vi "CRYGet Max Size.vi"(10 "Value Rows":i32[](array[numeric]), 11 "Curve Rows":i32[](array[numeric])) -> (3 "Max Size":i32)   [LabVIEW 2013]
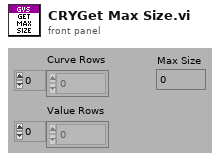
[diagram p1: front panel]
types:
  T1 = typedef "CRYData Cluster.ctl" = cluster{"Name":string, "Curve":cluster{"x":dbl, "y":dbl, "z":dbl}[], "X data":u16, "Y data":u16, "Z data":u16, "X axis":u16, "Y axis":u16, "Z axis":u16, "X unit":string, "Y unit":string, "Z unit":string, "X dB ref":dbl, "Y dB ref":dbl, "Z dB ref":dbl, "single val":bool, "protected":bool, "display X":bool, "display Y":bool, "display Z":bool, "Test Info":string, "Step No.":i32, "Plot Settings":cluster{"Color":u32, "Interpolation":u8, "Point Style":u8, "Line Style":u8, "Point Color":u32, "Line Width":u8, "Bar Plot Style":u8, "Fill To":i16}, "AutoProtect":bool}
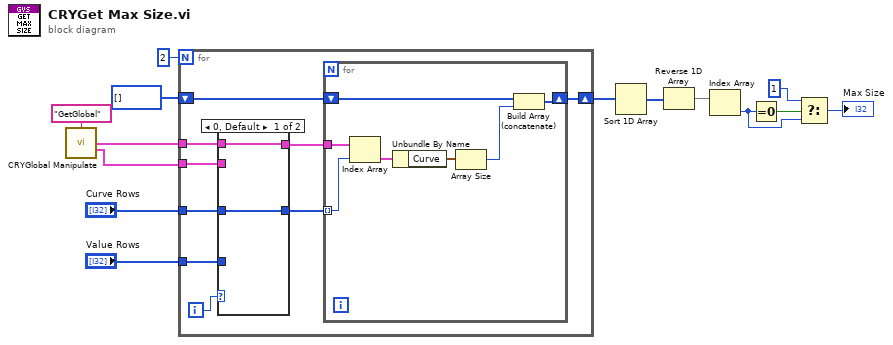
[diagram p0: block diagram]
diagram:
  n1 = call "CRYGlobal Manipulate.vi"("sAction"="GetGlobal") -> ("Curves Out"=w2:T1[], "Values Out"=w1:T1[])  [unwired: 8 in, 5 out]
  n2 = for {
    N: 2 -> [_]
    tunnel: w2 -> [w22]
    tunnel: w1 -> [w21]
    tunnel: "Curve Rows" -> [w20]
    tunnel: "Value Rows" -> [w19]
    shift-right: [w16] -> w10
    shift-left: i32[] [] ("Value Rows") -> [w15]
    i -> [w23]
    n3 = case shown="0, Default" w23 {
      tunnel: w22 -> [w32 _]
      tunnel: w21 -> [_ w34]
      tunnel: w20 -> [w31 _]
      tunnel: w19 -> [_ w33]
      tunnel: [w32 w34] -> w18
      tunnel: [w31 w33] -> w17
      frame 0, Default {
      }
      frame 1 {
      }
    }
    n4 = for {
      tunnel: w18 -> [w30]
      tunnel: w17 -> [w29] mode=indexing
      shift-right: [w24] -> w16
      shift-left: w15 -> [w26]
      n5 = Index Array(array=w30, index=w29) -> (element=w28:T1)
      n6 = Unbundle By Name(w28) -> ("Curve"=w27:cluster{"x":dbl, "y":dbl, "z":dbl}[])
      n7 = Array Size(array=w27) -> (size(s)=w25:i32)
      n8 = Build Array (concatenate)(w26, w25) -> (w24:i32[])
    }
  }
  n9 = Sort 1D Array(array=w10) -> (sorted array=w9:i32[])
  n10 = Reverse 1D Array(array=w9) -> (reversed array=w8:i32[])
  n11 = Index Array(array=w8) -> (element=w4:i32)  [unwired: 1 in]
  n12 = Equal To 0?(x=w4) -> (x = 0?=w7:bool)
  n13 = Select(t=1 ("Max Size"), s=w7, f=w4) -> (s? t:f=→"Max Size":i32)
